vi "Configure Current Limit Core.vi"(6 "behavior (regulate)":i32(ring) items=["Regulate", "Trip"], 8 "error in (no error)":errorcluster, 9 "limit (0.0 Amps)":dbl[unit] format="%^.2e", 10 "channel name (\"CHANNEL1\")":string="CHANNEL1", 11 "CS++DCPwr in":refnum<class "CS++DCPwr.lvclass">) -> (0 "error out":errorcluster, 3 "CS++DCPwr out":refnum<class "CS++DCPwr.lvclass">)   [LabVIEW 2016, in "CS++DCPwr.lvlib" / "CS++DCPwr.lvclass"]
doc: "This VI configures the current limit. You specify the output current limit value and the behavior of the power supply when the output current is greater than or equal to that value."
uses:
  CS++DCPwr.lvclass
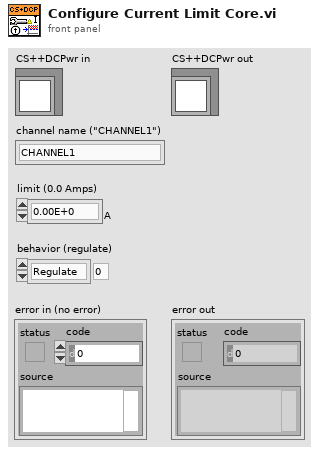
[diagram p1: front panel]
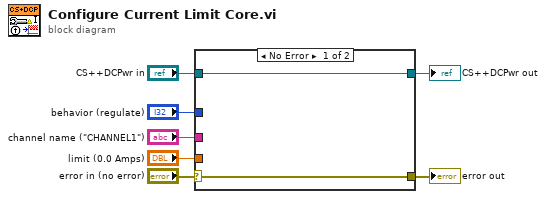
[diagram p0: block diagram]
diagram:
  n1 = case shown="No Error" "error in (no error)" {
    selector: "error in (no error)" -> [w8 w11]
    tunnel: [w8 w11] -> w6
    tunnel: [w9 w10] -> w4
    tunnel: "CS++DCPwr in" -> [w9 w10]
    tunnel: "channel name (\"CHANNEL1\")" -> [_ _]
    tunnel: "behavior (regulate)" -> [_ _]
    tunnel: "limit (0.0 Amps)" -> [_ _]
    frame No Error {
    }
    frame Error {
    }
  }
  "error out" <- w6
  "CS++DCPwr out" <- w4
